vi "InstrumentControlExercises_MichaelVasmerDavidWise.vi"() -> ()   [LabVIEW 2013]
doc: "This example shows how to configure a measurement and take a reading."
uses:
  Lab2/LabVIEW/Control2_MichaelVasmerDavidWise.ctl
  <instrlib>/Keithley 24XX/Public/Data/Read (Single Point).vi
  <vilib>/express/express arith-compare/Formula/XNode/ExpressFormulaBlockNode.xnode
  <instrlib>/Keithley 24XX/Keithley 24XX.lvlib
panel:
  in  "B Max":dbl
  out "State Machine State":T1=enum."Exit"
  in  "Sweep R(B)":bool
  in  "Steps":dbl
  out "Field too high error":string
  in  "Compliance  Level (0.1)":dbl=0.1
  out "Resistance":sgl
  out "Current":sgl
  out "Voltage":sgl
  in  "Enable Resistance Auto Range (T:Enable)":bool=TRUE
  in  "Enable Current Auto Range (T:Enable)":bool=TRUE
  in  "Enable Voltage Auto Range (T:Enable)":bool=TRUE
  in  "Resistance Manual Range (1.0)":dbl=1.0
  in  "Current Manual Range (1.0)":dbl=1.0
  in  "Voltage Manual Range (1.0)":dbl=1.0
  in  "Serial Configuration":T2={"Baud Rate"=9600, "Parity"=0, "Data Bits"=8, "Stop Bits"=10, "Flow Control"=0} {"Flow Control" items=["None", "XON/XOFF", "RTS/CTS", "XON/XOFF & RTS/CTS", "DTR/DSR", "XON/XOFF & DTR/DSR"]; "Stop Bits" items=["1.0"=10, "1.5"=15, "2.0"=20]; "Data Bits" items=["7"=7, "8"=8]; "Parity" items=["None", "Odd", "Even", "Mark", "Space"]; "Baud Rate" items=["300"=300, "600"=600, "1200"=1200, "2400"=2400, "4800"=4800, "9600"=9600, "19200"=19200]}
  in  "VISA resource name":refnum<visa-resource-name>
  # "Voltage Range Settings"
  # "Source Settings"
  # "Current Range Settings"
  # "Resistance Range Settings"
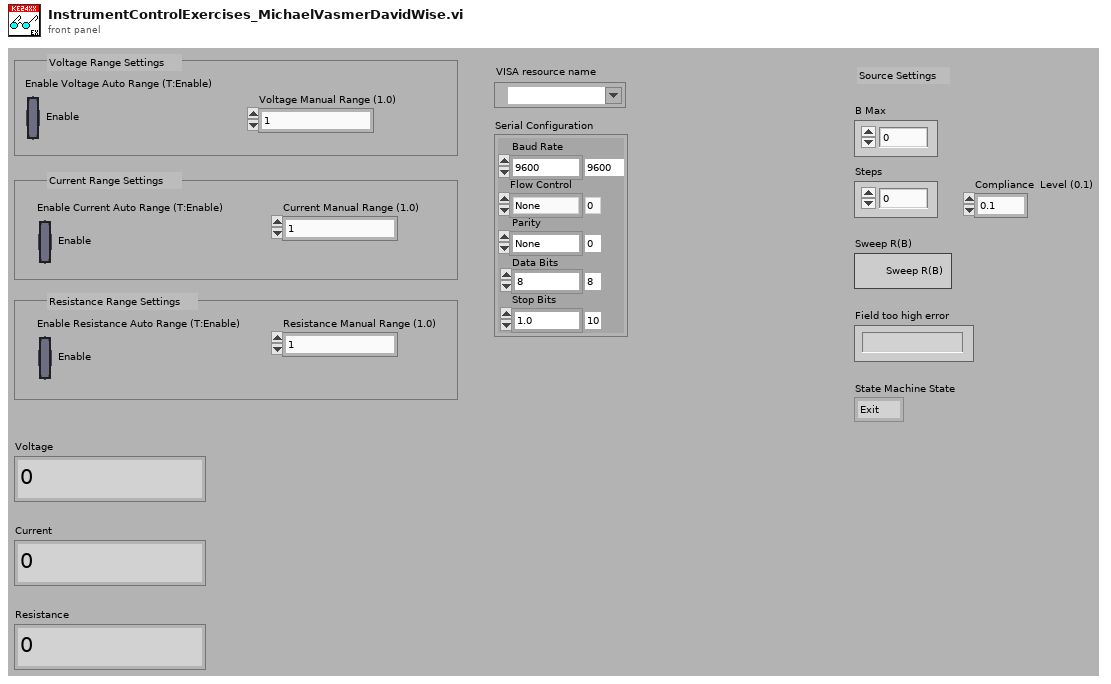
[diagram p1: front panel]
types:
  T1 = typedef "Control2_MichaelVasmerDavidWise.ctl" = enum16{"Increment", "Shutdown", "Idle", "Exit", "Read", "Set B", "Init"}
  T2 = cluster{"Baud Rate":u32, "Parity":u16, "Data Bits":u16, "Stop Bits":u16, "Flow Control":u16}
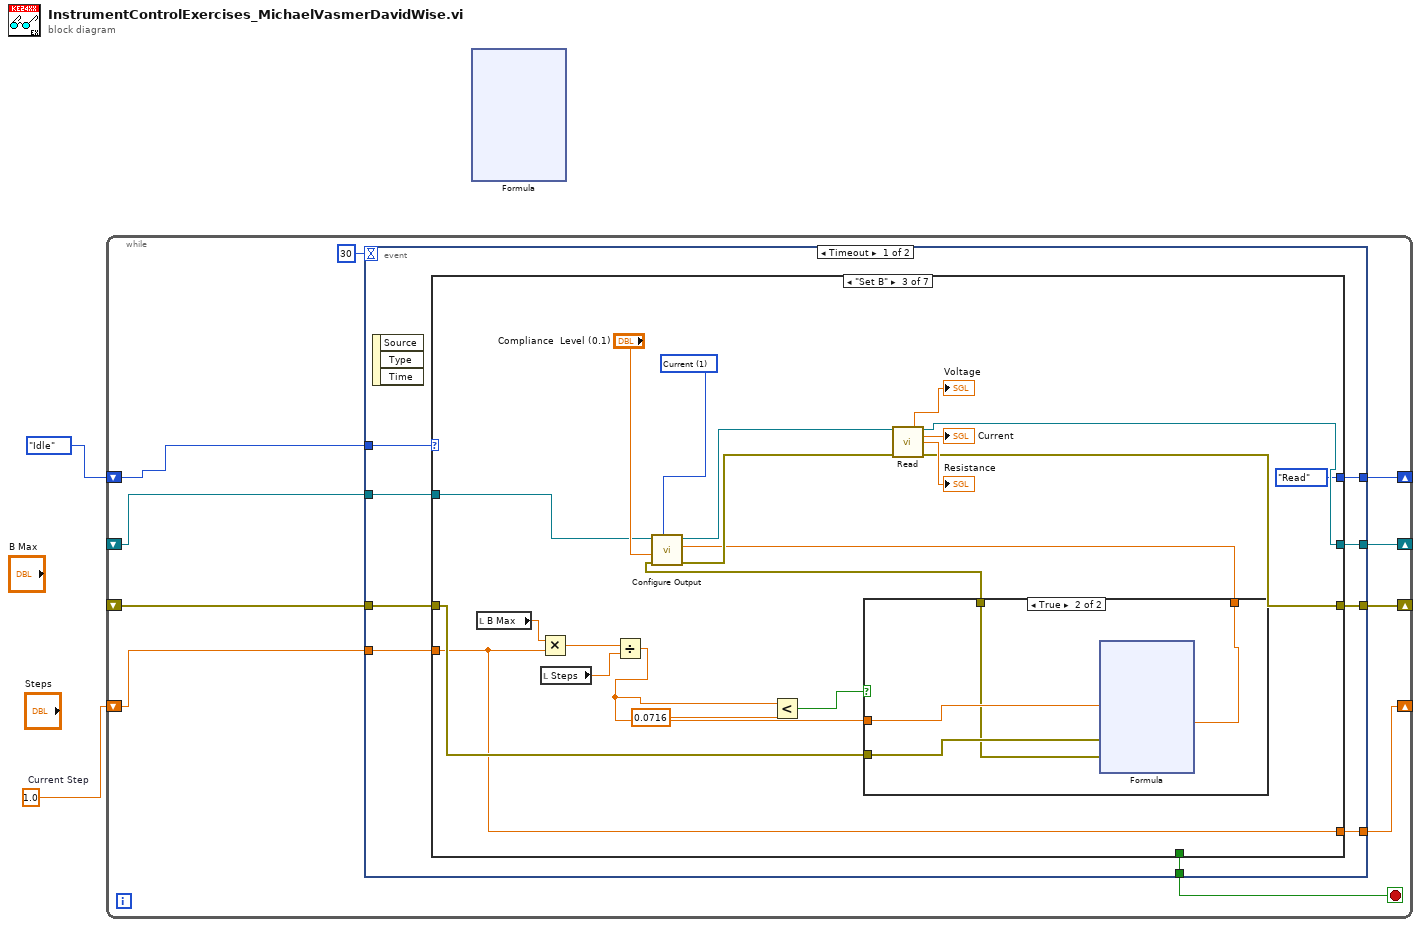
[diagram p0: block diagram]
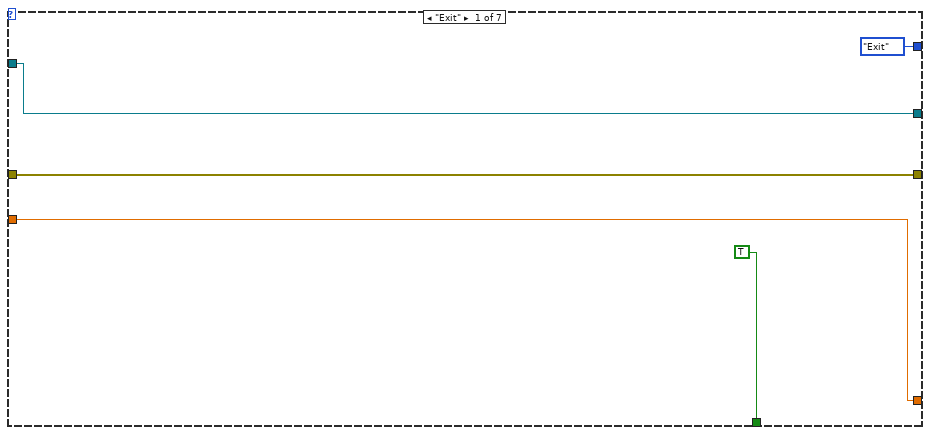
[diagram p2: hidden frame]
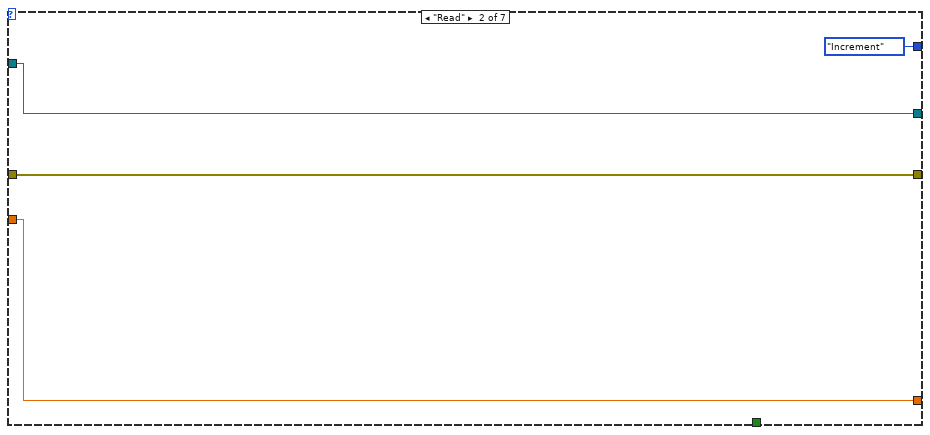
[diagram p3: hidden frame]
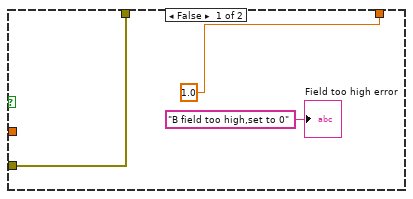
[diagram p4: hidden frame]
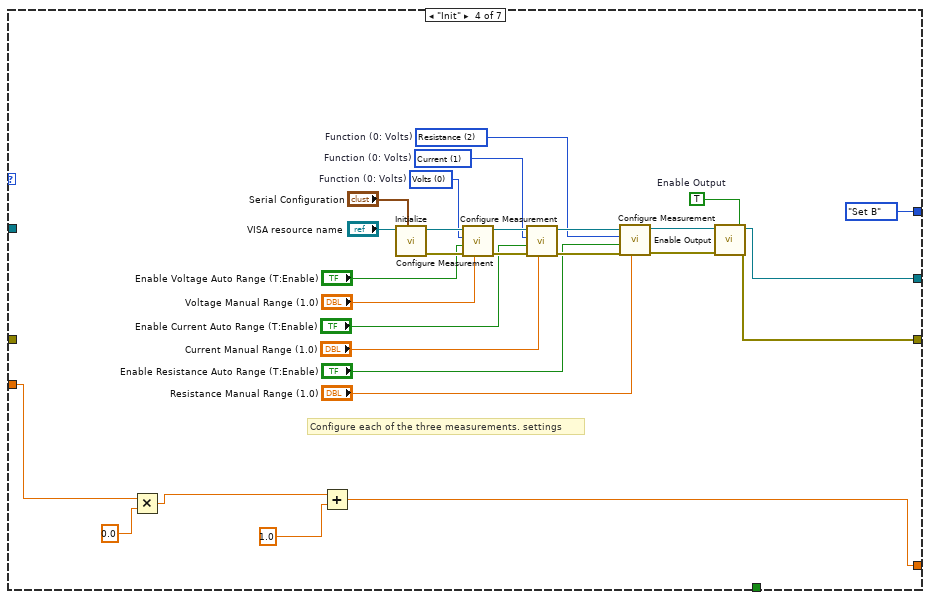
[diagram p5: hidden frame]
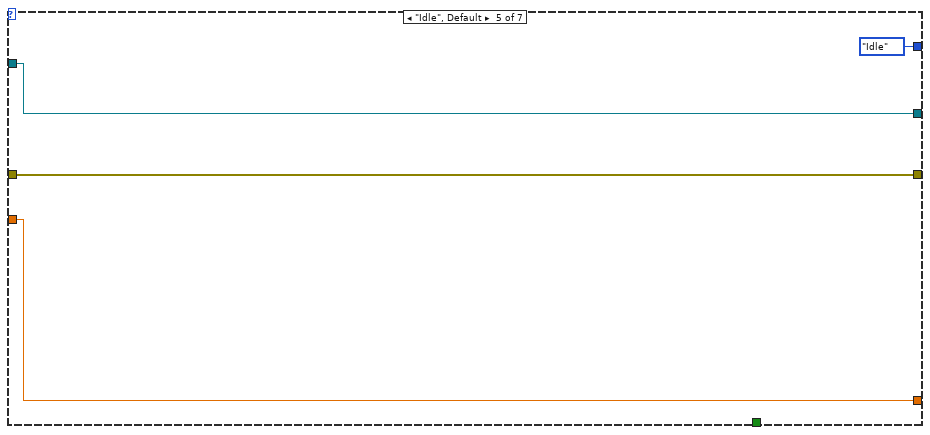
[diagram p6: hidden frame]
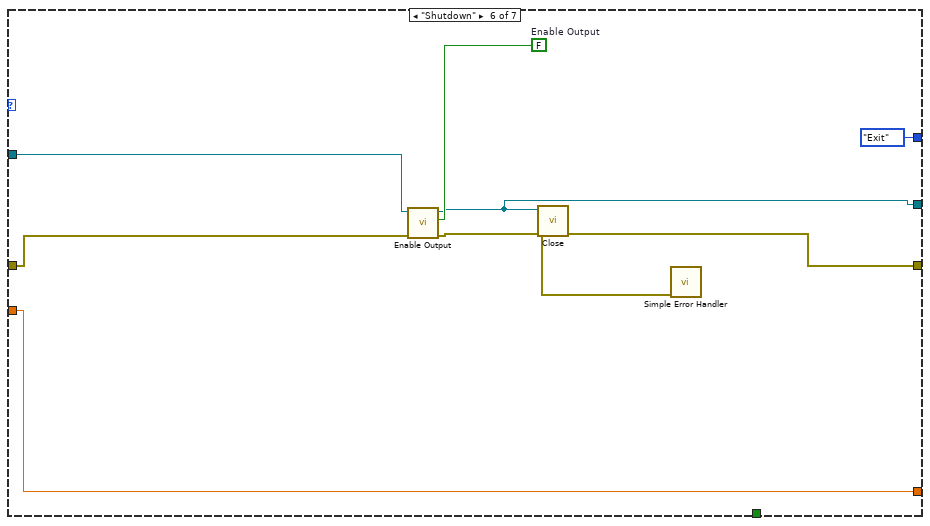
[diagram p7: hidden frame]
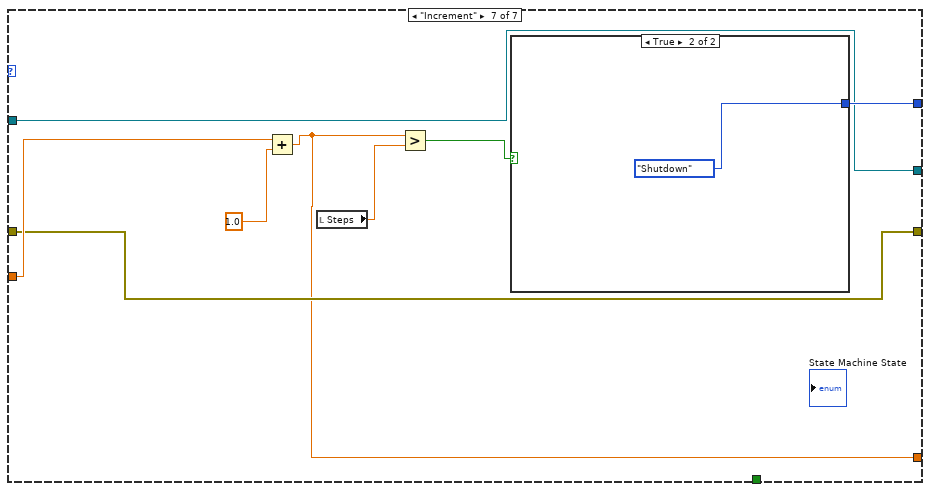
[diagram p8: hidden frame]
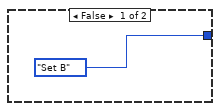
[diagram p9: hidden frame]
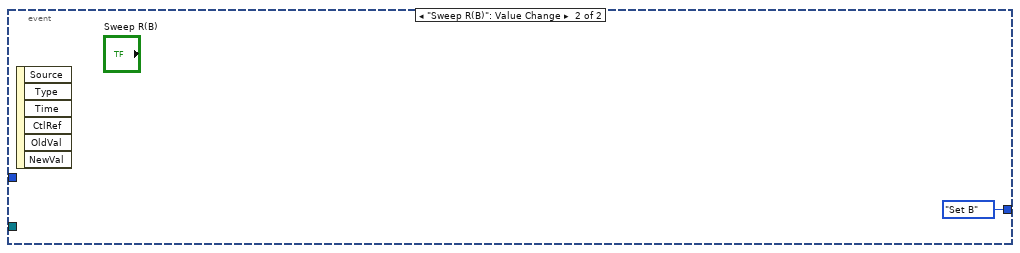
[diagram p10: hidden frame]
diagram:
  w1 = 1.0  # Current Step
  n1 = while {
    shift-right: [w11] -> _
    shift-left: Control2_MichaelVasmerDavidWise."Idle" -> [w12]
    shift-right: [w10] -> _
    shift-left: _ -> [w7]
    shift-right: [w9] -> _
    shift-left: _ -> [w6]
    shift-right: [w3] -> _
    shift-left: w1 -> [w4]
    stop <- w5 stop-if-true
    n2 = event shown="[0] Timeout" {
      selector: _ -> [_ _]
      dyn-events: _ -> [_ _]
      timeout: 30 -> [_ _]
      tunnel: w12 -> [w21 _]
      tunnel: [w20 Control2_MichaelVasmerDavidWise."Set B"] -> w11
      tunnel: [w19 _] -> w10
      tunnel: [w18 _] -> w9
      tunnel: w7 -> [w17 _]
      tunnel: w6 -> [w16 _]
      tunnel: [w15 _] -> w5
      tunnel: w4 -> [w14 _]
      tunnel: [w13 _] -> w3
      event Timeout {
        n3 = event-data() -> ()  [unwired: 1 in, 3 out]
        n4 = case shown="\"Set B\"" w21 {
          tunnel: [Control2_MichaelVasmerDavidWise."Exit" Control2_MichaelVasmerDavidWise."Increment" Control2_MichaelVasmerDavidWise."Read" Control2_MichaelVasmerDavidWise."Set B" Control2_MichaelVasmerDavidWise."Idle" Control2_MichaelVasmerDavidWise."Exit" w110] -> w20
          tunnel: [w25 w30 w44 w73 w96 w100 w109] -> w19
          tunnel: [w24 w29 w39 w72 w97 w102 w108] -> w18
          tunnel: w17 -> [w25 w30 w45 _ w96 w104 w109]
          tunnel: w16 -> [w24 w29 w41 _ w97 w103 w108]
          tunnel: [TRUE _ _ _ _ _ _] -> w15
          tunnel: w14 -> [w23 w28 w31 w71 w98 w99 w114]
          tunnel: [w23 w28 w31 w67 w98 w99 w107] -> w13
          frame "Exit" {
          }
          frame "Read" {
          }
          frame "Set B" {
            w43 = u16 1 items=["Voltage", "Current"] ("Source Mode  (0: Voltage)")
            n5 = local read "B Max"() -> (w35:dbl)
            n6 = Multiply(x=w35, y=w31) -> (x*y=w33:dbl)
            n7 = local read "Steps"() -> (w32:dbl)
            n8 = Divide(x=w33, y=w32) -> (x/y=w34:dbl)
            n9 = Less?(x=w34, y=0.0716 ("x")) -> (x < y?=w37:bool)
            n10 = case shown="True" w37 {
              tunnel: w34 -> [_ w58]
              tunnel: [1.0 ("x") w57] -> w42
              tunnel: w41 -> [w53 w56]
              tunnel: [w53 w55] -> w40
              frame False {
                "Field too high error" <- "B field too high,set to 0" ("String")
              }
              frame True {
                n11 = xnode "Formula"("X1"=w58, "error in (no error)"=w56) -> ("Result"=w57:dbl, "error out"=w55:errorcluster)
              }
            }
            n12 = call <instrlib>:"Configure Output.vi"("Source Mode  (0: Voltage)"=w43, "error in (no error)"=w40, "Compliance  Level (0.1)"="Compliance  Level (0.1)", "Output Level (0)"=w42, "VISA resource name"=w45) -> ("error out"=w46:errorcluster, "VISA resource name out"=w47:refnum<visa-resource-name>)  [unwired: 5 in]
            n13 = call-poly <instrlib>:"Read.vi"("VISA resource name"=w47, "error in (no error)"=w46) -> ("Voltage"=→"Voltage":sgl, "VISA resource name out"=w44:refnum<visa-resource-name>, "Current"=→"Current":sgl, "Resistance"=→"Resistance":sgl, "error out"=w39:errorcluster)  [unwired: 7 in, 2 out]
          }
          frame "Init" {
            w77 = TRUE  # Enable Output
            w84 = u16 2 items=["Volts", "Current", "Resistance"]  # Function (0: Volts)
            w85 = u16 1 items=["Volts", "Current", "Resistance"]  # Function (0: Volts)
            w86 = u16 0 items=["Volts", "Current", "Resistance"]  # Function (0: Volts)
            # "Configure each of the three measurements. settings"
            n14 = Multiply(x=w71, y=0.0 ("x")) -> (x*y=w70:dbl)
            n15 = Add(x=w70, y=1.0 ("x+y")) -> (x+y=w67:dbl)
            n16 = call <instrlib>:"Initialize.vi"("Serial Configuration"="Serial Configuration", "VISA resource name"="VISA resource name") -> ("error out"=w91:errorcluster, "VISA resource name out"=w92:refnum<visa-resource-name>)  [unwired: 8 in]
            n17 = call <instrlib>:"Configure Measurement.vi"("Manual Range (1.0)"="Voltage Manual Range (1.0)", "error in (no error)"=w91, "Enable Auto Range (T:Enable)"="Enable Voltage Auto Range (T:Enable)", "Function (0: Volts)"=w86, "VISA resource name"=w92) -> ("error out"=w89:errorcluster, "VISA resource name out"=w90:refnum<visa-resource-name>)  [unwired: 5 in]
            n18 = call <instrlib>:"Configure Measurement.vi"("Manual Range (1.0)"="Current Manual Range (1.0)", "error in (no error)"=w89, "Enable Auto Range (T:Enable)"="Enable Current Auto Range (T:Enable)", "Function (0: Volts)"=w85, "VISA resource name"=w90) -> ("error out"=w88:errorcluster, "VISA resource name out"=w87:refnum<visa-resource-name>)  [unwired: 5 in]
            n19 = call <instrlib>:"Configure Measurement.vi"("Manual Range (1.0)"="Resistance Manual Range (1.0)", "error in (no error)"=w88, "Enable Auto Range (T:Enable)"="Enable Resistance Auto Range (T:Enable)", "Function (0: Volts)"=w84, "VISA resource name"=w87) -> ("error out"=w75:errorcluster, "VISA resource name out"=w76:refnum<visa-resource-name>)  [unwired: 5 in]
            n20 = call <instrlib>:"Enable Output.vi"("error in (no error)"=w75, "Enable Output (T: Enable)"=w77, "VISA resource name"=w76) -> ("error out"=w72:errorcluster, "VISA resource name out"=w73:refnum<visa-resource-name>)  [unwired: 7 in]
          }
          frame "Idle", Default {
          }
          frame "Shutdown" {
            w106 = FALSE  # Enable Output
            n21 = call <instrlib>:"Enable Output.vi"("error in (no error)"=w103, "Enable Output (T: Enable)"=w106, "VISA resource name"=w104) -> ("error out"=w105:errorcluster, "VISA resource name out"=w100:refnum<visa-resource-name>)  [unwired: 7 in]
            n22 = call <instrlib>:"Close.vi"("error in (no error)"=w105, "VISA resource name"=w100) -> ("error out"=w102:errorcluster)  [unwired: 9 in]
            n23 = call <vilib>:"Simple Error Handler.vi"("error in (no error)"=w102) -> ()  [unwired: 4 in, 5 out]
          }
          frame "Increment" {
            n24 = Add(x=w114, y=1.0 ("x")) -> (x+y=w107:dbl)
            n25 = local read "Steps"() -> (w112:dbl)
            n26 = Greater?(x=w107, y=w112) -> (0:w111:bool)
            n27 = case shown="True" w111 {
              tunnel: [Control2_MichaelVasmerDavidWise."Set B" Control2_MichaelVasmerDavidWise."Shutdown"] -> w110
              frame False {
              }
              frame True {
              }
            }
          }
        }
      }
      event "Sweep R(B)": Value Change {
        n28 = event-data() -> ()  [unwired: 1 in, 6 out]
      }
    }
  }
  n29 = xnode "Formula"() -> ()  [unwired: 2 in, 2 out]
